vi "JSON DIDDLE.vi"() -> ()   [LabVIEW 2016, in "Control Experiment.lvclass"]
uses:
  Control Experiment.lvclass
  Typedefs/Control Experiment JSON--cluster.ctl
  Transport/Typedefs/Lockin_Vsg JSON--Cluster.ctl
  Transport/Transport.lvclass
  SweepControl/Typedefs/Cluster - ScanParamters.ctl
  SweepControl/SweepControl.lvclass
  SweepControl/Typedefs/ScanParamters.ctl
  SweepControl/Typedefs/Enum - Action.ctl
  SweepControl/Typedefs/Enum - Priority.ctl
  SweepControl/Typedefs/Cluster - ScanControl.ctl
  SweepControl/Typedefs/ScanControl.ctl
  SweepControl/Typedefs/Enum - Experiments.ctl
  SweepControl/Typedefs/Sweep Control JSON--Cluster.ctl
  <userlib>/LevyLab/Lockin-Multichannel/Lockin.DAQ/Typedefs/Sweep Pattern--Enum.ctl
  <userlib>/LevyLab/Lockin-Multichannel/Lockin.DAQ/Lockin.DAQ.lvclass
  <userlib>/LevyLab/Lockin-Multichannel/Instrument.Lockinl.UI/Typedefs/Sweep Channel--Cluster.ctl
  <userlib>/LevyLab/Lockin-Multichannel/Instrument.Lockinl.UI/Instrument.Lockin.UI.lvclass
  <userlib>/LevyLab/Lockin-Multichannel/Lockin.DAQ/Typedefs/Sweep Configuration--Cluster.ctl
  <userlib>/LevyLab/Krohn Hite 7008/typedefs/Input Configuration-Enum.ctl
  <userlib>/LevyLab/Krohn Hite 7008/Instrument.KH7008.lvclass
  <userlib>/LevyLab/Krohn Hite 7008/typedefs/Coupling-Enum.ctl
  <userlib>/LevyLab/Krohn Hite 7008/typedefs/Shunt-Enum.ctl
  <userlib>/LevyLab/Krohn Hite 7008/typedefs/Filter-Enum.ctl
  <userlib>/LevyLab/Krohn Hite 7008/typedefs/Gain-Enum.ctl
  <userlib>/LevyLab/Krohn Hite 7008/typedefs/Channel-Enum.ctl
  <userlib>/LevyLab/Krohn Hite 7008/typedefs/SetAll-Cluster.ctl
  <userlib>/LevyLab/Krohn Hite 7008/typedefs/SetAll-Array.ctl
  <userlib>/LevyLab/Lockin-Multichannel/Instrument.Lockinl.UI/Typedefs/REF Channel--Cluster.ctl
  <userlib>/LevyLab/Lockin-Multichannel/Lockin.DAQ/Typedefs/REF-cluster.ctl
  <userlib>/LevyLab/Lockin-Multichannel/Lockin.DAQ/Typedefs/Function-enum.ctl
  <userlib>/LevyLab/Lockin-Multichannel/Instrument.Lockinl.UI/Typedefs/AO Channel--Cluster.ctl
  <userlib>/LevyLab/Lockin-Multichannel/Lockin.DAQ/Typedefs/AO-cluster.ctl
  Typedefs/Wiring Description--cluster.ctl
  Typedefs/Instrument--enum.ctl
  Typedefs/Experiment Description--cluster.ctl
  SweepControl/Typedefs/Continuous B Sweep JSON--Cluster.ctl
  <vilib>/addons/_JKI.lib/Serialization/JSON/JKI JSON Serialization.lvlib
panel:
  in  "Enum":T1(ring)=enum."Lockin Sweep"
  out "JSON String":string
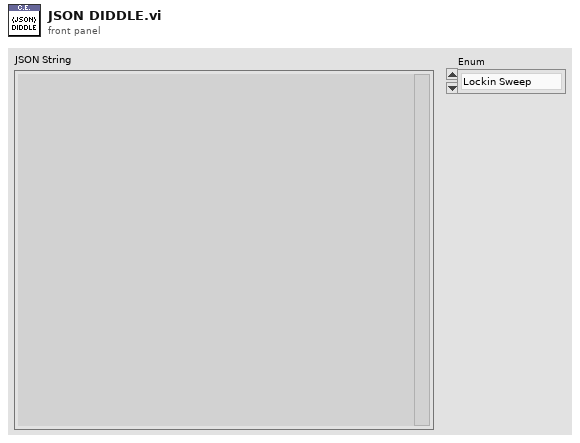
[diagram p1: front panel]
types:
  T1 = enum16{"C.E.", "Sweep Control", "Continuous B", "Lockin Vsg", "Lockin Sweep"}
  T2 = typedef "SweepControl.lvclass/Continuous B Sweep JSON--Cluster.ctl" = cluster{"Continuous B Sweep":cluster{"Experiment":T3, "B field values":dbl[]}, "Experiment Description":T4, "Wiring Configuration":T6, "Lockin":cluster{"Channels: AO":T7, "Channels: Lockin":T10}, "Krohn Hite":cluster{"Channel Setting":T12}}
  T3 = typedef "SweepControl.lvclass/Enum - Experiments.ctl" = enum16{"IV", "IV_Fast", "THz_DelayLine", "Lockin_Vsg", "Lockin_Sweep", "Lockin_Time", "AI WFM time", "Lockin (experimental)"}
  T4 = typedef "Control Experiment.lvclass/Experiment Description--cluster.ctl" = cluster{"User":string, "Device":string, "Device Path":path, "Device Description":string, "Experiment Path":path, "Experiment Description":string, "Instrument":T5, "Device Description (JSON)":string, "Experiment Description (JSON)":string, "Comments":string, "Sweep":cluster{"key":string, "value":variant}[]}
  T5 = typedef "Control Experiment.lvclass/Instrument--enum.ctl" = enum16{"----- AFM/EBL -----", "AGILENT", "CYPHER", "Gemini2", "JEOL", "MFP3D", "----- Cryostat -----", "CF900", "DR200", "MNK", "PPMS 1", "PPMS 2", "PPMS 3", "----- Optics -----", "THz 1", "THz 2"}
  T6 = typedef "Control Experiment.lvclass/Wiring Description--cluster.ctl" = cluster{"AI":cluster{"Channel":u32, "Gain":dbl}, "Device":cluster{"Electrode":string, "Label":string, "Type":string}, "KH":cluster{"Channel":string, "Configuration":string, "Gain":u32, "Shunt Resistor":u32}, "AO":cluster{"Channel":u32, "Gain":dbl}}[]
  T7 = typedef "Lockin.DAQ.lvclass/AO-cluster.ctl" = T8[]
  T8 = typedef "Instrument.Lockin.UI.lvclass/AO Channel--Cluster.ctl" = cluster{"Enable?":bool, "Channel":i32, "Amplitude":dbl, "Offset":dbl, "Frequency":dbl, "Phase":dbl, "Function":T9, "Sweeping?":bool}
  T9 = typedef "Lockin.DAQ.lvclass/Function-enum.ctl" = enum16{"Sine", "Triangle", "Square"}
  T10 = typedef "Lockin.DAQ.lvclass/REF-cluster.ctl" = T11[]
  T11 = typedef "Instrument.Lockin.UI.lvclass/REF Channel--Cluster.ctl" = cluster{"Enable?":bool, "Channel":i32, "Frequency":dbl, "Phase":dbl, "TC":dbl, "Order":i32}
  T12 = typedef "Instrument.KH7008.lvclass/SetAll-Array.ctl" = T13[]
  T13 = typedef "Instrument.KH7008.lvclass/SetAll-Cluster.ctl" = cluster{"Channel":T14, "Gain":T15, "Bandwidth Filter":T16, "Shunt Resistor":T17, "Coupling":T18, "Input Config":T19}
  T14 = typedef "Instrument.KH7008.lvclass/Channel-Enum.ctl" = enum16{"Channel 1", "Channel 2", "Channel 3", "Channel 4", "Channel 5", "Channel 6", "Channel 7", "Channel 8"}
  T15 = typedef "Instrument.KH7008.lvclass/Gain-Enum.ctl" = enum16{"1x", "10x", "100x", "1000x"}
  T16 = typedef "Instrument.KH7008.lvclass/Filter-Enum.ctl" = enum16{"OFF", "ON"}
  T17 = typedef "Instrument.KH7008.lvclass/Shunt-Enum.ctl" = enum16{"Open", "50 Ohms", "500 Ohms", "5k Ohms", "50k Ohms", "10M Ohm"}
  T18 = typedef "Instrument.KH7008.lvclass/Coupling-Enum.ctl" = enum16{"AC", "DC"}
  T19 = typedef "Instrument.KH7008.lvclass/Input Configuration-Enum.ctl" = enum16{"Ground", "SE+ (-gnd)", "SE- (+gnd)", "Differential"}
  T20 = typedef "Lockin.DAQ.lvclass/Sweep Configuration--Cluster.ctl" = cluster{"Sweep Time (s)":dbl, "Initial Wait (s)":dbl, "Return to Start":bool, "Channels":T21[]}
  T21 = typedef "Instrument.Lockin.UI.lvclass/Sweep Channel--Cluster.ctl" = cluster{"End":dbl, "Start":dbl, "Channel":u16, "Pattern":T22}
  T22 = typedef "Lockin.DAQ.lvclass/Sweep Pattern--Enum.ctl" = enum16{"Ramp /", "Ramp /\\", "Smooth Ramp _/", "Smooth Ramp _/\\_", "Frequency"}
  T23 = typedef "SweepControl.lvclass/Sweep Control JSON--Cluster.ctl" = cluster{"Experiment":T3, "Repeat Experiment":i32, "Scan control":T24, "Scan parameters":T28}
  T24 = typedef "SweepControl.lvclass/ScanControl.ctl" = T25[]
  T25 = typedef "SweepControl.lvclass/Cluster - ScanControl.ctl" = cluster{"Priority":T26, "Scan name":T27}
  T26 = typedef "SweepControl.lvclass/Enum - Priority.ctl" = enum16{"Priority 0", "Priority 1", "Priority 2", "Priority 3", "Priority 4", "Priority 5"}
  T27 = typedef "SweepControl.lvclass/Enum - Action.ctl" = enum16{"OFF", "time", "Lockin Amplitude", "Lockin Frequency", "Lockin Bias", "Delay", "Strain", "DAQ Bias", "Magnet Field", "Temperature", "MW f1", "MW f2", "MW Amplitude1", "MW Amplitude2"}
  T28 = typedef "SweepControl.lvclass/ScanParamters.ctl" = T29[]
  T29 = typedef "SweepControl.lvclass/Cluster - ScanParamters.ctl" = cluster{"Start":dbl, "End":dbl, "Step":dbl, "Rate":dbl, "Waveform type":enum16{"linear", "triangle", "power"}, "wait (ms or K)":dbl, "Address":string, "channel":i32}
  T30 = typedef "Transport.lvclass/Lockin_Vsg JSON--Cluster.ctl" = cluster{"Vsg Values":dbl[]}
  T31 = typedef "Control Experiment.lvclass/Control Experiment JSON--cluster.ctl" = cluster{"Device":cluster{"Device":string, "User":string, "Time":string, "Computer Name":string}, "Wiring":cluster{"Lockin Ch":u32[], "KH Electrodes":string[], "KH Labels":string[], "Other Electrodes":string[], "Other Labels":string[]}}
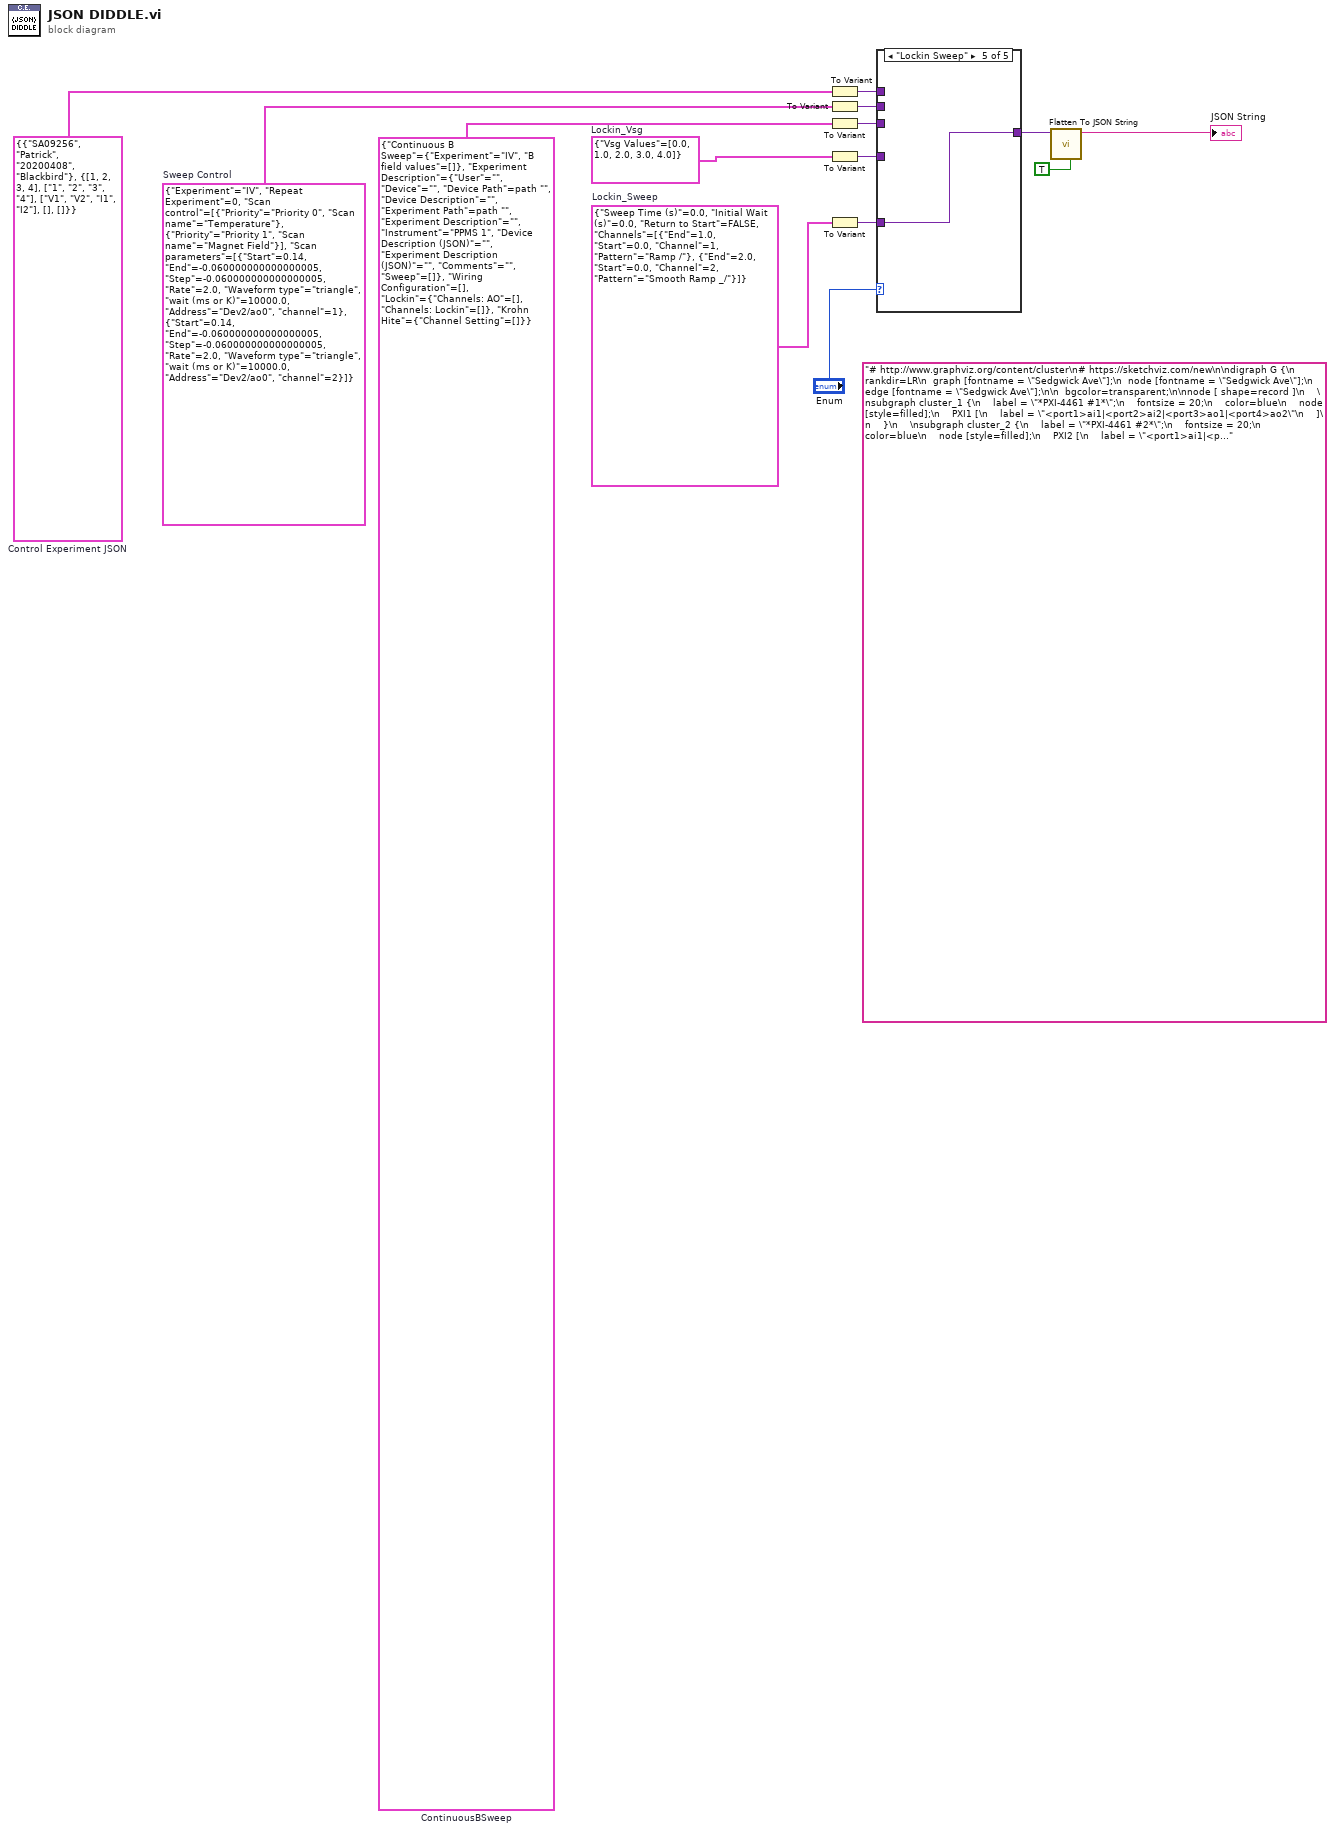
[diagram p0: block diagram]
diagram:
  (unwired) "# http://www.graphviz.org/content/cluster\n# https://sketchviz.com/new\n\ndigraph G {\n    rankdir=LR\n  graph [fontname = \"Sedgwick Ave\"];\n  node [fontname = \"Sedgwick Ave\"];\n  edge [fontname = \"Sedgwick Ave\"];\n\n  bgcolor=transparent;\n\nnode [ shape=record ]\n    \nsubgraph cluster_1 {\n    label = \"*PXI-4461 #1*\";\n    fontsize = 20;\n    color=blue\n    node [style=filled];\n    PXI1 [\n    label = \"<port1>ai1|<port2>ai2|<port3>ao1|<port4>ao2\"\n    ]\n    }\n    \nsubgraph cluster_2 {\n    label = \"*PXI-4461 #2*\";\n    fontsize = 20;\n    color=blue\n    node [style=filled];\n    PXI2 [\n    label = \"<port1>ai1|<port2>ai2|<port3>ao1|<port4>ao2\"\n    ]\n    }\n    \nsubgraph cluster_3 {\n    label = \"*PXI-4461 #3*\";\n    fontsize = 20;\n    color=blue\n    node [style=filled];\n    PXI3 [\n    label = \"<port1>ai1|<port2>ai2|<port3>ao1|<port4>ao2\"\n    ]\n    }\n    \nsubgraph cluster_4 {\n    label = \"*PXI-4461 #4*\";\n    fontsize = 20;\n    color=blue\n    node [style=filled];\n    PXI4 [\n    label = \"<port1>ai1|<port2>ai2|<port3>ao1|<port4>ao2\"\n    ]\n    }\n    \nsubgraph cluster_5 {\n    label = \"*KH7008 #1*\";\n    fontsize = 20;\n    color=blue\n    node [style=filled];\n    KH1 [\n        label = \"<port1>In+|<port2>In-|<port3>Out\"\n        ]\n    KH2 [\n        label = \"<port1>In+|<port2>In-|<port3>Out\"\n        ]\n    KH3 [\n        label = \"<port1>In+|<port2>In-|<port3>Out\"\n        ]\n    KH4 [\n        label = \"<port1>In+|<port2>In-|<port3>Out\"\n        ]\n    KH5 [\n        label = \"<port1>In+|<port2>In-|<port3>Out\"\n        ]\n    KH6 [\n        label = \"<port1>In+|<port2>In-|<port3>Out\"\n        ]\n    KH7 [\n        label = \"<port1>In+|<port2>In-|<port3>Out\"\n        ]\n    KH8 [\n        label = \"<port1>In+|<port2>In-|<port3>Out\"\n        ]\n    \n}\n\nsubgraph cluster_6 {\n    1, 2, 3, 4, 5, 6, 7, 8, 9, 10, 11, 12, 13, 14, 15, 16, 17, 18, 19, 20, 21, 22, 23, 24, 25, 26, 27, 28\n};\n    \n    \nPXI1:port3 -> KH1:port2\nPXI1:port4 -> KH2:port2\nPXI2:port3 -> KH3:port2\nPXI2:port4 -> KH4:port2\nPXI3:port3 -> KH5:port2\nPXI3:port4 -> KH6:port2\nPXI4:port3 -> KH7:port2\nPXI4:port4 -> KH8:port2\nKH1:port3 -> PXI1:port1\nKH2:port3 -> PXI1:port2\nKH3:port3 -> PXI2:port1\nKH4:port3 -> PXI2:port2\nKH5:port3 -> PXI3:port1\nKH6:port3 -> PXI3:port2\nKH7:port3 -> PXI4:port1\nKH8:port3 -> PXI4:port2\n\n}"
  w9 = T2 {"Continuous B Sweep"={"Experiment"=enum."IV", "B field values"=[]}, "Experiment Description"={"User"="", "Device"="", "Device Path"=path "", "Device Description"="", "Experiment Path"=path "", "Experiment Description"="", "Instrument"=enum."PPMS 1", "Device Description (JSON)"="", "Experiment Description (JSON)"="", "Comments"="", "Sweep"=[]}, "Wiring Configuration"=[], "Lockin"={"Channels: AO"=[], "Channels: Lockin"=[]}, "Krohn Hite"={"Channel Setting"=[]}}  # ContinuousBSweep
  w4 = T20 {"Sweep Time (s)"=0.0, "Initial Wait (s)"=0.0, "Return to Start"=FALSE, "Channels"=[{"End"=1.0, "Start"=0.0, "Channel"=1, "Pattern"=enum."Ramp /"}, {"End"=2.0, "Start"=0.0, "Channel"=2, "Pattern"=enum."Smooth Ramp _/"}]}  # Lockin_Sweep
  w12 = T23 {"Experiment"=enum."IV", "Repeat Experiment"=0, "Scan control"=[{"Priority"=enum."Priority 0", "Scan name"=enum."Temperature"}, {"Priority"=enum."Priority 1", "Scan name"=enum."Magnet Field"}], "Scan parameters"=[{"Start"=0.14, "End"=-0.060000000000000005, "Step"=-0.060000000000000005, "Rate"=2.0, "Waveform type"=enum."triangle", "wait (ms or K)"=10000.0, "Address"="Dev2/ao0", "channel"=1}, {"Start"=0.14, "End"=-0.060000000000000005, "Step"=-0.060000000000000005, "Rate"=2.0, "Waveform type"=enum."triangle", "wait (ms or K)"=10000.0, "Address"="Dev2/ao0", "channel"=2}]}  # Sweep Control
  w3 = T30 {"Vsg Values"=[0.0, 1.0, 2.0, 3.0, 4.0]}  # Lockin_Vsg
  w13 = T31 {"Device"={"Device"="SA09256", "User"="Patrick", "Time"="20200408", "Computer Name"="Blackbird"}, "Wiring"={"Lockin Ch"=[1, 2, 3, 4], "KH Electrodes"=["1", "2", "3", "4"], "KH Labels"=["V1", "V2", "I1", "I2"], "Other Electrodes"=[], "Other Labels"=[]}}  # Control Experiment JSON
  n1 = To Variant(anything=w13) -> (Variant=w10:variant)
  n2 = To Variant(anything=w12) -> (Variant=w11:variant)
  n3 = To Variant(anything=w9) -> (Variant=w7:variant)
  n4 = To Variant(anything=w3) -> (Variant=w6:variant)
  n5 = To Variant(anything=w4) -> (Variant=w5:variant)
  n6 = case shown="\"Lockin Sweep\"" "Enum" {
    tunnel: [w15 w16 w17 w18 w19] -> w2
    tunnel: w10 -> [w15 _ _ _ _]
    tunnel: w11 -> [_ w16 _ _ _]
    tunnel: w7 -> [_ _ w17 _ _]
    tunnel: w6 -> [_ _ _ w18 _]
    tunnel: w5 -> [_ _ _ _ w19]
    frame "C.E." {
    }
    frame "Sweep Control" {
    }
    frame "Continuous B" {
    }
    frame "Lockin Vsg" {
    }
    frame "Lockin Sweep" {
    }
  }
  n7 = call <vilib>:"Flatten To JSON String.vi"("Enums As String (F)"=TRUE, "Variant"=w2) -> ("JSON String"=→"JSON String":string)  [unwired: 8 in, 1 out]
